vi "xy_stack_global.vi"() -> ()   [LabVIEW 2016]
panel:
  out "Write protection":bool
  out "Scanning":refnum<user-event>
  in  "FOV Frame (um)":dbl(ring)=0.471281296023564 items=["4x4 µm"=0.01860032550569635, "8x8 µm"=0.0372006510113927, "16x16 µm"=0.0744013020227854, "32x32 µm"=0.1488026040455708, "64x64 µm"=0.2976052080911416, "128x128 µm"=0.5952104161822832, "256x256 µm"=1.1904208323645664, "512x512 µm"=2.380841664729133, "1024x1024 µm"=4.761683329458266, "0x0"=0.0]
  in  "Number of pixels Frame":i32(ring)=128 items=["8x8"=8, "16x16"=16, "32x32"=32, "64x64"=64, "128x128"=128, "256x256"=256, "512x512"=512, "1024x1024"=1024, "optimal"=1014]
  in  "Warning Limits":dbl[][](array[numeric])
  out "event ImgUpdate":refnum<user-event>
  out "stage delay long":dbl=1.0
  out "stage delay short":dbl=1.0
  out "requested y-position":dbl=35000.0
  out "requested x-position":dbl=35000.0
  out "Move to Y":bool
  out "Move to X":bool
  out "# steps Y":u16=20 step=1 format="%#.0f"
  out "Y-Maximum":dbl=35000.0 format="%#.2f"
  out "Y-Minimum":dbl=35000.0 format="%#.2f"
  out "Step size Y":dbl=1.0 min=0.0
  out "Y-Position":sgl format="%.2f"
  out "# steps X":u16=20 step=1 format="%#.0f"
  out "X-Maximum":dbl=35000.0 format="%#.2f"
  out "X-Minimum":dbl=35000.0 format="%#.2f"
  out "Step size X":dbl=1.0 min=0.0
  out "X-Position":sgl format="%.2f"
  # "!!! Arbitrary, assumes Objective is centrally)\n(Objective Might leave Microscope Slide/Petri Dish)"
  # "Mosaicing info from Beamscanner"
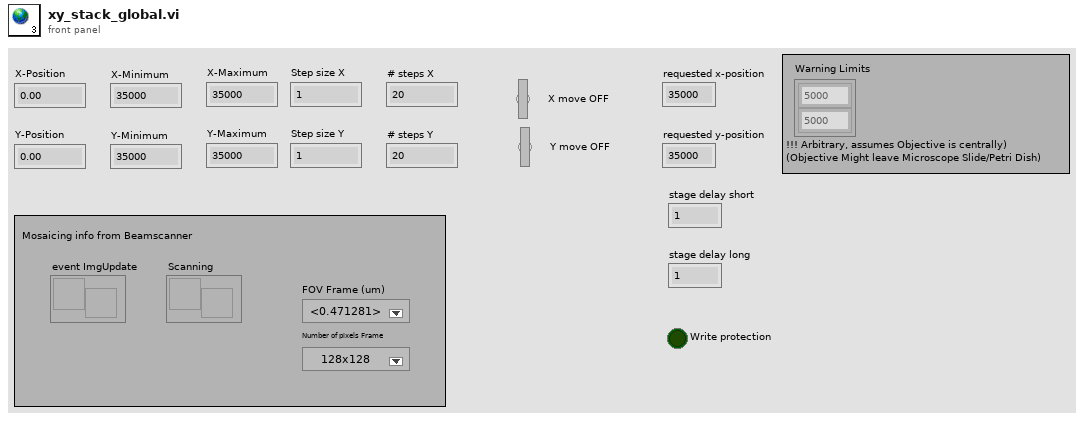
[diagram p1: front panel]
diagram:
